vi "PID Integral Action (DBL Array).vi"(4 "output range":cluster{"output high":dbl, "output low":dbl}[](array[cluster]) {"output low" format="%.2f"; "output high" format="%.2f"}, 5 "error":dbl[](array[numeric]) format="%.2f", 6 "dt (min)":dbl format="%.3f", 7 "proportional action":dbl[](array[numeric]) format="%.2f", 8 "initialize (F)":bool, 9 "derivative action":dbl[](array[numeric]) format="%.2f", 10 "PID gains":T1(array[cluster]) {"derivative time (Td, min)" format="%.3f"; "integral time (Ti, min)" format="%.3f"; "proportional gain (Kc)" format="%.3f"}, 11 "Ki":dbl[](array[numeric]) format="%.2f") -> (3 "output":dbl[](array[numeric]) format="%.2f")   [LabVIEW 2017, in "NI_PID_pid.lvlib"]
uses:
  <vilib>/addons/control/pid/NI_PID_pid.lvlib
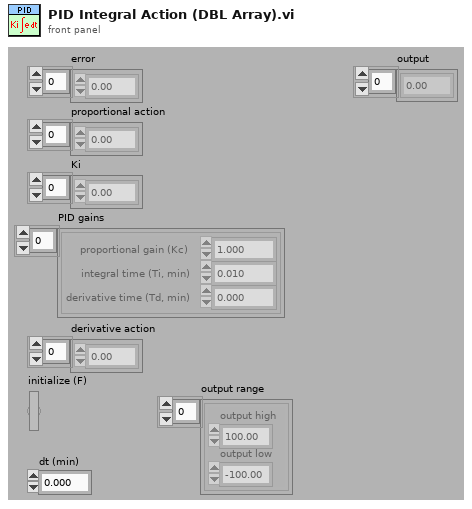
[diagram p1: front panel]
types:
  T1 = cluster{"proportional gain (Kc)":dbl, "integral time (Ti, min)":dbl, "derivative time (Td, min)":dbl}[]
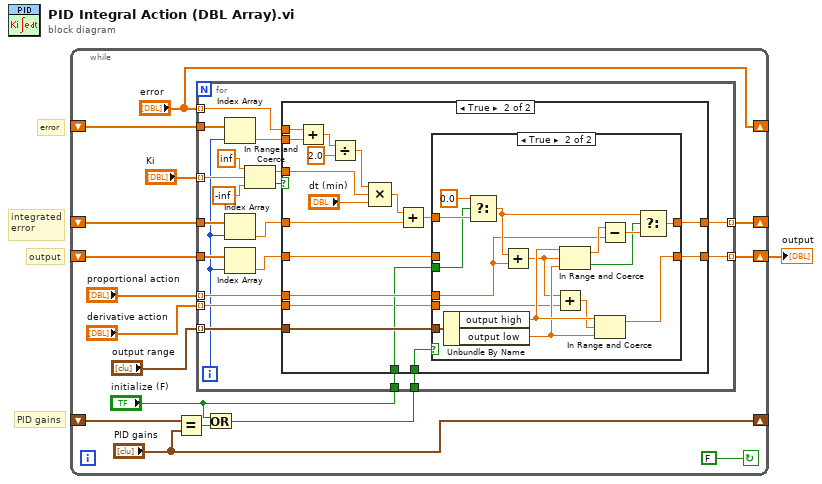
[diagram p0: block diagram]
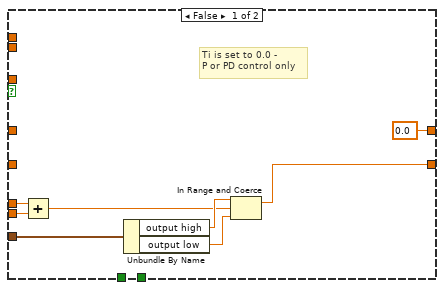
[diagram p2: hidden frame]
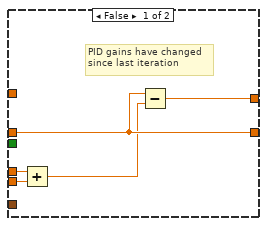
[diagram p3: hidden frame]
diagram:
  # "PID gains"
  # "output"
  # "integrated\nerror"
  # "error"
  n1 = while {
    shift-left: _ -> [w14]
    shift-right: [w13] -> w1
    shift-left: _ -> [w17]
    shift-right: ["error"] -> _
    shift-left: _ -> [w16]
    shift-right: [w15] -> _
    shift-left: _ -> [w9]
    shift-right: ["PID gains"] -> _
    stop <- FALSE continue-if-true
    n2 = Equal?(x=w9, y="PID gains") -> (x = y?=w8:bool)
    n3 = Or(x="initialize (F)", y=w8) -> (x .or. y?=w6:bool)
    n4 = for {
      tunnel: w17 -> [w19]
      tunnel: w16 -> [w22]
      tunnel: [w37] -> w15 mode=indexing
      tunnel: "proportional action" -> [w36] mode=indexing
      tunnel: w14 -> [w33]
      tunnel: [w32] -> w13 mode=indexing
      tunnel: "error" -> [w30] mode=indexing
      tunnel: "Ki" -> [w29] mode=indexing
      tunnel: "initialize (F)" -> [w28]
      tunnel: w6 -> [w27]
      tunnel: "output range" -> [w26] mode=indexing
      tunnel: "derivative action" -> [w25] mode=indexing
      i -> [w18]
      n5 = Index Array(array=w19, index=w18) -> (element=w20:dbl)
      n6 = Index Array(array=w22, index=w18) -> (element=w21:dbl)
      n7 = Index Array(array=w33, index=w18) -> (element=w24:dbl)
      n8 = In Range and Coerce(upper limit=inf, x=w29, lower limit=-inf) -> (coerced(x)=w31:dbl, In Range?=w34:bool)
      n9 = case shown="True" w34 {
        tunnel: w30 -> [_ w62]
        tunnel: w20 -> [_ w63]
        tunnel: w21 -> [_ w57]
        tunnel: [0.0 ("t") w52] -> w37
        tunnel: w31 -> [_ w50]
        tunnel: w36 -> [w39 w55]
        tunnel: [w45 w51] -> w32
        tunnel: w26 -> [w44 w53]
        tunnel: w24 -> [_ w54]
        tunnel: w28 -> [_ w48]
        tunnel: w27 -> [_ w47]
        tunnel: w25 -> [w40 w46]
        frame False {
          # "Ti is set to 0.0 -\nP or PD control only"
          n10 = Add(x=w39, y=w40) -> (x+y=w38:dbl)
          n11 = Unbundle By Name(w44) -> ("output high"=w43:dbl, "output low"=w42:dbl)
          n12 = In Range and Coerce(upper limit=w43, x=w38, lower limit=w42) -> (coerced(x)=w45:dbl)  [unwired: 1 out]
        }
        frame True {
          n13 = Add(x=w62, y=w63) -> (x+y=w60:dbl)
          n14 = Divide(x=w60, y=2.0) -> (x/y=w59:dbl)
          n15 = Compound Arithmetic op=MULTIPLY(w59, w50, "dt (min)") -> (w58:dbl)
          n16 = Add(x=w58, y=w57) -> (x+y=w56:dbl)
          n17 = case shown="True" w47 {
            tunnel: w56 -> [_ w75]
            tunnel: w55 -> [w65 w73]
            tunnel: w54 -> [w68 _]
            tunnel: w48 -> [_ w74]
            tunnel: w53 -> [_ w70]
            tunnel: [w67 w69] -> w52
            tunnel: [w68 w71] -> w51
            tunnel: w46 -> [w66 w72]
            frame False {
              # "PID gains have changed\nsince last iteration"
              n18 = Add(x=w65, y=w66) -> (x+y=w64:dbl)
              n19 = Subtract(x=w68, y=w64) -> (x-y=w67:dbl)
            }
            frame True {
              n20 = Unbundle By Name(w70) -> ("output high"=w82:dbl, "output low"=w81:dbl)
              n21 = Select(t=0.0, s=w74, f=w75) -> (s? t:f=w78:dbl)
              n22 = Add(x=w78, y=w73) -> (x+y=w77:dbl)
              n23 = Add(x=w77, y=w72) -> (x+y=w76:dbl)
              n24 = In Range and Coerce(upper limit=w82, x=w77, lower limit=w81) -> (coerced(x)=w80:dbl, In Range?=w79:bool)
              n25 = In Range and Coerce(upper limit=w82, x=w76, lower limit=w81) -> (coerced(x)=w71:dbl)  [unwired: 1 out]
              n26 = Subtract(x=w80, y=w73) -> (x-y=w83:dbl)
              n27 = Select(t=w78, s=w79, f=w83) -> (s? t:f=w69:dbl)
            }
          }
        }
      }
    }
  }
  "output" <- w1
